vi "driveForwardFast Command.vi"(10 "Data":string[](array[string]), 11 "Robot dev revs":T1={"Drive"={"Drive Actuaters"={"Motor devRevs"={"Left Side Motors"={"Motor 1 devRev"={"DeviceStatus"={"status"=FALSE, "code"=0, "source"=""}, "Type"=enum."PWM", "PWM"={"Digital Module"=enum."Digital Module 1", "PWM Channel"=enum."PWM 1", "DeadBand"={"Name"="", "maxPositivePwm"=0, "minPositivePwm"=0, "centerPwm"=0, "maxNegativePwm"=0, "minNegativePwm"=0, "angularRange"=0}}, "CAN"={"Device Number"=0, "Control Mode"=enum."Percent VBus", "Semaphore"=refnum, "Max Vout"=0.0}, "Invert"=FALSE, "TransformRef"=refnum, "InvTransformRef"=refnum}, "Motor 2 devRev"={"DeviceStatus"={"status"=FALSE, "code"=0, "source"=""}, "Type"=enum."PWM", "PWM"={"Digital Module"=enum."Digital Module 1", "PWM Channel"=enum."PWM 1", "DeadBand"={"Name"="", "maxPositivePwm"=0, "minPositivePwm"=0, "centerPwm"=0, "maxNegativePwm"=0, "minNegativePwm"=0, "angularRange"=0}}, "CAN"={"Device Number"=0, "Control Mode"=enum."Percent VBus", "Semaphore"=refnum, "Max Vout"=0.0}, "Invert"=FALSE, "TransformRef"=refnum, "InvTransformRef"=refnum}, "Motor 3 devRev"={"DeviceStatus"={"status"=FALSE, "code"=0, "source"=""}, "Type"=enum."PWM", "PWM"={"Digital Module"=enum."Digital Module 1", "PWM Channel"=enum."PWM 1", "DeadBand"={"Name"="", "maxPositivePwm"=0, "minPositivePwm"=0, "centerPwm"=0, "maxNegativePwm"=0, "minNegativePwm"=0, "angularRange"=0}}, "CAN"={"Device Number"=0, "Control Mode"=enum."Percent VBus", "Semaphore"=refnum, "Max Vout"=0.0}, "Invert"=FALSE, "TransformRef"=refnum, "InvTransformRef"=refnum}}, "Right Side Motors"={"Motor 1 devRev"={"DeviceStatus"={"status"=FALSE, "code"=0, "source"=""}, "Type"=enum."PWM", "PWM"={"Digital Module"=enum."Digital Module 1", "PWM Channel"=enum."PWM 1", "DeadBand"={"Name"="", "maxPositivePwm"=0, "minPositivePwm"=0, "centerPwm"=0, "maxNegativePwm"=0, "minNegativePwm"=0, "angularRange"=0}}, "CAN"={"Device Number"=0, "Control Mode"=enum."Percent VBus", "Semaphore"=refnum, "Max Vout"=0.0}, "Invert"=FALSE, "TransformRef"=refnum, "InvTransformRef"=refnum}, "Motor 2 devRev"={"DeviceStatus"={"status"=FALSE, "code"=0, "source"=""}, "Type"=enum."PWM", "PWM"={"Digital Module"=enum."Digital Module 1", "PWM Channel"=enum."PWM 1", "DeadBand"={"Name"="", "maxPositivePwm"=0, "minPositivePwm"=0, "centerPwm"=0, "maxNegativePwm"=0, "minNegativePwm"=0, "angularRange"=0}}, "CAN"={"Device Number"=0, "Control Mode"=enum."Percent VBus", "Semaphore"=refnum, "Max Vout"=0.0}, "Invert"=FALSE, "TransformRef"=refnum, "InvTransformRef"=refnum}, "Motor 3 devRev"={"DeviceStatus"={"status"=FALSE, "code"=0, "source"=""}, "Type"=enum."PWM", "PWM"={"Digital Module"=enum."Digital Module 1", "PWM Channel"=enum."PWM 1", "DeadBand"={"Name"="", "maxPositivePwm"=0, "minPositivePwm"=0, "centerPwm"=0, "maxNegativePwm"=0, "minNegativePwm"=0, "angularRange"=0}}, "CAN"={"Device Number"=0, "Control Mode"=enum."Percent VBus", "Semaphore"=refnum, "Max Vout"=0.0}, "Invert"=FALSE, "TransformRef"=refnum, "InvTransformRef"=refnum}}, "dev Status"={"status"=FALSE, "code"=0, "source"=""}}, "SolenoidDevRef"={"DevStatus"={"status"=FALSE, "code"=0, "source"=""}, "Solenoid Module"=enum."Solenoid Module 1", "Forward Solenoid Channel"=enum."Solenoid 1", "Reverse Solenoid Channel"=enum."Solenoid 1"}}, "Drive Sensor data"={"Encoders"={"Right Encoder"={"DevStatus"={"status"=FALSE, "code"=0, "source"=""}, "EncoderIndex"=enum."Enc 0", "CounterIndex"=enum."Ctr 0", "DistancePerCount"=0.0, "Decoding Type"=enum."1x"}}, "GyroDevRef"={"DevStatus"={"status"=FALSE, "code"=0, "source"=""}, "Analog Module"=enum."Analog Module 1", "Analog Channel"=enum."AI 1", "Offset"=0.0, "Gain (VoltsPerDegree/Second)"=0.0}, "Last commanded Angle"=0.0}}, "Catapult devrevs"={"MotorControlDeviceRef"={"DeviceStatus"={"status"=FALSE, "code"=0, "source"=""}, "Type"=enum."PWM", "PWM"={"Digital Module"=enum."Digital Module 1", "PWM Channel"=enum."PWM 1", "DeadBand"={"Name"="", "maxPositivePwm"=0, "minPositivePwm"=0, "centerPwm"=0, "maxNegativePwm"=0, "minNegativePwm"=0, "angularRange"=0}}, "CAN"={"Device Number"=0, "Control Mode"=enum."Percent VBus", "Semaphore"=refnum, "Max Vout"=0.0}, "Invert"=FALSE, "TransformRef"=refnum, "InvTransformRef"=refnum}, "SolenoidDevRef"={"DevStatus"={"status"=FALSE, "code"=0, "source"=""}, "Solenoid Module"=enum."Solenoid Module 1", "Forward Solenoid Channel"=enum."Solenoid 1", "Reverse Solenoid Channel"=enum."Solenoid 1"}, "first limit switch"={"DevStatus"={"status"=FALSE, "code"=0, "source"=""}, "DIO Channel"=enum."DIO 1", "Digital Module"=enum."Digital Module 1"}, "second limit switch"={"DevStatus"={"status"=FALSE, "code"=0, "source"=""}, "DIO Channel"=enum."DIO 1", "Digital Module"=enum."Digital Module 1"}}, "Drive Joystick"={"Device"=enum."USB 1"}, "Operator Joystick"={"Device"=enum."USB 1"}, "roller devrevs"={"SolenoidDevRef"={"DevStatus"={"status"=FALSE, "code"=0, "source"=""}, "Solenoid Module"=enum."Solenoid Module 1", "Forward Solenoid Channel"=enum."Solenoid 1", "Reverse Solenoid Channel"=enum."Solenoid 1"}, "MotorControlDeviceRef"={"DeviceStatus"={"status"=FALSE, "code"=0, "source"=""}, "Type"=enum."PWM", "PWM"={"Digital Module"=enum."Digital Module 1", "PWM Channel"=enum."PWM 1", "DeadBand"={"Name"="", "maxPositivePwm"=0, "minPositivePwm"=0, "centerPwm"=0, "maxNegativePwm"=0, "minNegativePwm"=0, "angularRange"=0}}, "CAN"={"Device Number"=0, "Control Mode"=enum."Percent VBus", "Semaphore"=refnum, "Max Vout"=0.0}, "Invert"=FALSE, "TransformRef"=refnum, "InvTransformRef"=refnum}, "DigitalInputDevRef"={"DevStatus"={"status"=FALSE, "code"=0, "source"=""}, "DIO Channel"=enum."Invalid", "Digital Module"=enum."Digital Module 1"}}, "Puncher devrevs"={"SolenoidDevRef"={"DevStatus"={"status"=FALSE, "code"=0, "source"=""}, "Solenoid Module"=enum."Solenoid Module 1", "Forward Solenoid Channel"=enum."Solenoid 1", "Reverse Solenoid Channel"=enum."Solenoid 1"}, "DigitalInputDevRef"={"DevStatus"={"status"=FALSE, "code"=0, "source"=""}, "DIO Channel"=enum."DIO 1", "Digital Module"=enum."Digital Module 1"}}}) -> (3 "Robot dev revs out":T1={"Drive"={"Drive Actuaters"={"Motor devRevs"={"Left Side Motors"={"Motor 1 devRev"={"DeviceStatus"={"status"=FALSE, "code"=0, "source"=""}, "Type"=enum."PWM", "PWM"={"Digital Module"=enum."Digital Module 1", "PWM Channel"=enum."PWM 1", "DeadBand"={"Name"="", "maxPositivePwm"=0, "minPositivePwm"=0, "centerPwm"=0, "maxNegativePwm"=0, "minNegativePwm"=0, "angularRange"=0}}, "CAN"={"Device Number"=0, "Control Mode"=enum."Percent VBus", "Semaphore"=refnum, "Max Vout"=0.0}, "Invert"=FALSE, "TransformRef"=refnum, "InvTransformRef"=refnum}, "Motor 2 devRev"={"DeviceStatus"={"status"=FALSE, "code"=0, "source"=""}, "Type"=enum."PWM", "PWM"={"Digital Module"=enum."Digital Module 1", "PWM Channel"=enum."PWM 1", "DeadBand"={"Name"="", "maxPositivePwm"=0, "minPositivePwm"=0, "centerPwm"=0, "maxNegativePwm"=0, "minNegativePwm"=0, "angularRange"=0}}, "CAN"={"Device Number"=0, "Control Mode"=enum."Percent VBus", "Semaphore"=refnum, "Max Vout"=0.0}, "Invert"=FALSE, "TransformRef"=refnum, "InvTransformRef"=refnum}, "Motor 3 devRev"={"DeviceStatus"={"status"=FALSE, "code"=0, "source"=""}, "Type"=enum."PWM", "PWM"={"Digital Module"=enum."Digital Module 1", "PWM Channel"=enum."PWM 1", "DeadBand"={"Name"="", "maxPositivePwm"=0, "minPositivePwm"=0, "centerPwm"=0, "maxNegativePwm"=0, "minNegativePwm"=0, "angularRange"=0}}, "CAN"={"Device Number"=0, "Control Mode"=enum."Percent VBus", "Semaphore"=refnum, "Max Vout"=0.0}, "Invert"=FALSE, "TransformRef"=refnum, "InvTransformRef"=refnum}}, "Right Side Motors"={"Motor 1 devRev"={"DeviceStatus"={"status"=FALSE, "code"=0, "source"=""}, "Type"=enum."PWM", "PWM"={"Digital Module"=enum."Digital Module 1", "PWM Channel"=enum."PWM 1", "DeadBand"={"Name"="", "maxPositivePwm"=0, "minPositivePwm"=0, "centerPwm"=0, "maxNegativePwm"=0, "minNegativePwm"=0, "angularRange"=0}}, "CAN"={"Device Number"=0, "Control Mode"=enum."Percent VBus", "Semaphore"=refnum, "Max Vout"=0.0}, "Invert"=FALSE, "TransformRef"=refnum, "InvTransformRef"=refnum}, "Motor 2 devRev"={"DeviceStatus"={"status"=FALSE, "code"=0, "source"=""}, "Type"=enum."PWM", "PWM"={"Digital Module"=enum."Digital Module 1", "PWM Channel"=enum."PWM 1", "DeadBand"={"Name"="", "maxPositivePwm"=0, "minPositivePwm"=0, "centerPwm"=0, "maxNegativePwm"=0, "minNegativePwm"=0, "angularRange"=0}}, "CAN"={"Device Number"=0, "Control Mode"=enum."Percent VBus", "Semaphore"=refnum, "Max Vout"=0.0}, "Invert"=FALSE, "TransformRef"=refnum, "InvTransformRef"=refnum}, "Motor 3 devRev"={"DeviceStatus"={"status"=FALSE, "code"=0, "source"=""}, "Type"=enum."PWM", "PWM"={"Digital Module"=enum."Digital Module 1", "PWM Channel"=enum."PWM 1", "DeadBand"={"Name"="", "maxPositivePwm"=0, "minPositivePwm"=0, "centerPwm"=0, "maxNegativePwm"=0, "minNegativePwm"=0, "angularRange"=0}}, "CAN"={"Device Number"=0, "Control Mode"=enum."Percent VBus", "Semaphore"=refnum, "Max Vout"=0.0}, "Invert"=FALSE, "TransformRef"=refnum, "InvTransformRef"=refnum}}, "dev Status"={"status"=FALSE, "code"=0, "source"=""}}, "SolenoidDevRef"={"DevStatus"={"status"=FALSE, "code"=0, "source"=""}, "Solenoid Module"=enum."Solenoid Module 1", "Forward Solenoid Channel"=enum."Solenoid 1", "Reverse Solenoid Channel"=enum."Solenoid 1"}}, "Drive Sensor data"={"Encoders"={"Right Encoder"={"DevStatus"={"status"=FALSE, "code"=0, "source"=""}, "EncoderIndex"=enum."Enc 0", "CounterIndex"=enum."Ctr 0", "DistancePerCount"=0.0, "Decoding Type"=enum."1x"}}, "GyroDevRef"={"DevStatus"={"status"=FALSE, "code"=0, "source"=""}, "Analog Module"=enum."Analog Module 1", "Analog Channel"=enum."AI 1", "Offset"=0.0, "Gain (VoltsPerDegree/Second)"=0.0}, "Last commanded Angle"=0.0}}, "Catapult devrevs"={"MotorControlDeviceRef"={"DeviceStatus"={"status"=FALSE, "code"=0, "source"=""}, "Type"=enum."PWM", "PWM"={"Digital Module"=enum."Digital Module 1", "PWM Channel"=enum."PWM 1", "DeadBand"={"Name"="", "maxPositivePwm"=0, "minPositivePwm"=0, "centerPwm"=0, "maxNegativePwm"=0, "minNegativePwm"=0, "angularRange"=0}}, "CAN"={"Device Number"=0, "Control Mode"=enum."Percent VBus", "Semaphore"=refnum, "Max Vout"=0.0}, "Invert"=FALSE, "TransformRef"=refnum, "InvTransformRef"=refnum}, "SolenoidDevRef"={"DevStatus"={"status"=FALSE, "code"=0, "source"=""}, "Solenoid Module"=enum."Solenoid Module 1", "Forward Solenoid Channel"=enum."Solenoid 1", "Reverse Solenoid Channel"=enum."Solenoid 1"}, "first limit switch"={"DevStatus"={"status"=FALSE, "code"=0, "source"=""}, "DIO Channel"=enum."DIO 1", "Digital Module"=enum."Digital Module 1"}, "second limit switch"={"DevStatus"={"status"=FALSE, "code"=0, "source"=""}, "DIO Channel"=enum."DIO 1", "Digital Module"=enum."Digital Module 1"}}, "Drive Joystick"={"Device"=enum."USB 1"}, "Operator Joystick"={"Device"=enum."USB 1"}, "roller devrevs"={"SolenoidDevRef"={"DevStatus"={"status"=FALSE, "code"=0, "source"=""}, "Solenoid Module"=enum."Solenoid Module 1", "Forward Solenoid Channel"=enum."Solenoid 1", "Reverse Solenoid Channel"=enum."Solenoid 1"}, "MotorControlDeviceRef"={"DeviceStatus"={"status"=FALSE, "code"=0, "source"=""}, "Type"=enum."PWM", "PWM"={"Digital Module"=enum."Digital Module 1", "PWM Channel"=enum."PWM 1", "DeadBand"={"Name"="", "maxPositivePwm"=0, "minPositivePwm"=0, "centerPwm"=0, "maxNegativePwm"=0, "minNegativePwm"=0, "angularRange"=0}}, "CAN"={"Device Number"=0, "Control Mode"=enum."Percent VBus", "Semaphore"=refnum, "Max Vout"=0.0}, "Invert"=FALSE, "TransformRef"=refnum, "InvTransformRef"=refnum}, "DigitalInputDevRef"={"DevStatus"={"status"=FALSE, "code"=0, "source"=""}, "DIO Channel"=enum."Invalid", "Digital Module"=enum."Digital Module 1"}}, "Puncher devrevs"={"SolenoidDevRef"={"DevStatus"={"status"=FALSE, "code"=0, "source"=""}, "Solenoid Module"=enum."Solenoid Module 1", "Forward Solenoid Channel"=enum."Solenoid 1", "Reverse Solenoid Channel"=enum."Solenoid 1"}, "DigitalInputDevRef"={"DevStatus"={"status"=FALSE, "code"=0, "source"=""}, "DIO Channel"=enum."DIO 1", "Digital Module"=enum."Digital Module 1"}}})   [LabVIEW 2013]
uses:
  Robot dev revs.ctl
  Drive Code/Drive typedef.ctl
  Drive Code/Drive Motors Typedef.ctl
  Drive Code/GearBox Typedef.ctl
  <vilib>/Rock Robotics/WPI/MotorControl/WPI_MotorControlDeviceRef.ctl
  <vilib>/Rock Robotics/SystemInterfaces/Typedef/FPGA_TypedefDigitalModule.ctl
  <vilib>/Rock Robotics/SystemInterfaces/DIO/FPGA_DIOPWMChannel.ctl
  <vilib>/Rock Robotics/WPI/PWM/WPI_PWMDeadband.ctl
  <vilib>/Rock Robotics/WPI/CAN/Jaguar/SubVIs/WPI_CANJaguar_ControlMode.ctl
  <vilib>/Rock Robotics/WPI/PWM/WPI_PWMTransform_ConPane.ctl
  <vilib>/Rock Robotics/WPI/Solenoid/WPI_SolenoidDevRef.ctl
  <vilib>/Rock Robotics/SystemInterfaces/Typedef/FPGA_TypedefSolenoidModule.ctl
  <vilib>/Rock Robotics/WPI/Solenoid/WPI_SolenoidChannel.ctl
  Drive Code/Drive Sensor Typedef.ctl
  <vilib>/Rock Robotics/WPI/Encoder/WPI_EncoderDevRef.ctl
  <vilib>/Rock Robotics/SystemInterfaces/Encoder/FPGA_EncoderIdx.ctl
  <vilib>/Rock Robotics/SystemInterfaces/Counter/FPGA_CounterCtrSystemIndex.ctl
  <vilib>/Rock Robotics/WPI/Encoder/WPI_EncoderType.ctl
  <vilib>/Rock Robotics/WPI/Gyro/WPI_GyroDevRef.ctl
  <vilib>/Rock Robotics/SystemInterfaces/Typedef/FPGA_TypedefAnalogModule.ctl
  <vilib>/Rock Robotics/SystemInterfaces/AI/FPGA_AIChannel.ctl
  catapult code/catapult type def.ctl
  <vilib>/Rock Robotics/WPI/DigitalInput/WPI_DigitalInputDevRef.ctl
  <vilib>/Rock Robotics/SystemInterfaces/DIO/FPGA_DIOChannel.ctl
  <vilib>/Rock Robotics/WPI/Joystick/WPI_JoystickDevRef.ctl
  <vilib>/Rock Robotics/WPI/Joystick/WPI_JoystickDeviceEnum.ctl
  Roller V2/roller typedef.ctl
  Puncher/Puncher type.ctl
  Drive Auto/All Auto Drive constants.ctl
  Drive Auto/Drive auto constants.ctl
  Drive Code/Auto Transmission Code/All Shifter Constants.ctl
  Drive Code/Auto Transmission Code/Shift Constants.ctl
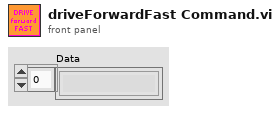
[diagram p1: front panel]
types:
  T1 = typedef "Robot dev revs.ctl" = cluster{"Drive":T2, "Catapult devrevs":T23, "Drive Joystick":T26, "Operator Joystick":T26, "roller devrevs":T28, "Puncher devrevs":T29}
  T2 = typedef "Drive typedef.ctl" = cluster{"Drive Actuaters":cluster{"Motor devRevs":T3, "SolenoidDevRef":T12}, "Drive Sensor data":T15}
  T3 = typedef "Drive Motors Typedef.ctl" = cluster{"Left Side Motors":T4, "Right Side Motors":T4, "dev Status":errorcluster}
  T4 = typedef "GearBox Typedef.ctl" = cluster{"Motor 1 devRev":T5, "Motor 2 devRev":T5, "Motor 3 devRev":T5}
  T5 = typedef "WPI_MotorControlDeviceRef.ctl" = cluster{"DeviceStatus":errorcluster, "Type":enum16{"PWM", "CAN"}, "PWM":cluster{"Digital Module":T6, "PWM Channel":T7, "DeadBand":T8}, "CAN":cluster{"Device Number":u8, "Control Mode":T9, "Semaphore":T10, "Max Vout":dbl}, "Invert":bool, "TransformRef":T11, "InvTransformRef":T11}
  T6 = typedef "FPGA_TypedefDigitalModule.ctl" = enum16{"Digital Module 1", "Digital Module 2"}
  T7 = typedef "FPGA_DIOPWMChannel.ctl" = enum8{"PWM 1", "PWM 2", "PWM 3", "PWM 4", "PWM 5", "PWM 6", "PWM 7", "PWM 8", "PWM 9", "PWM 10", "Invalid"}
  T8 = typedef "WPI_PWMDeadband.ctl" = cluster{"Name":string, "maxPositivePwm":i32, "minPositivePwm":i32, "centerPwm":i32, "maxNegativePwm":i32, "minNegativePwm":i32, "angularRange":u16}
  T9 = typedef "WPI_CANJaguar_ControlMode.ctl" = enum8{"Percent VBus", "Current", "Speed", "Position", "Voltage"}
  T10 = typedef "Semaphore RefNum" = refnum<k1>
  T11 = typedef "WPI_PWMTransform_ConPane.ctl" = refnum<vi>
  T12 = typedef "WPI_SolenoidDevRef.ctl" = cluster{"DevStatus":errorcluster, "Solenoid Module":T13, "Forward Solenoid Channel":T14, "Reverse Solenoid Channel":T14}
  T13 = typedef "FPGA_TypedefSolenoidModule.ctl" = enum16{"Solenoid Module 1", "Solenoid Module 2"}
  T14 = typedef "WPI_SolenoidChannel.ctl" = enum8{"Solenoid 1", "Solenoid 2", "Solenoid 3", "Solenoid 4", "Solenoid 5", "Solenoid 6", "Solenoid 7", "Solenoid 8", "Invalid"}
  T15 = typedef "Drive Sensor Typedef.ctl" = cluster{"Encoders":cluster{"Right Encoder":T16}, "GyroDevRef":T20, "Last commanded Angle":dbl}
  T16 = typedef "WPI_EncoderDevRef.ctl" = cluster{"DevStatus":errorcluster, "EncoderIndex":T17, "CounterIndex":T18, "DistancePerCount":dbl, "Decoding Type":T19}
  T17 = typedef "FPGA_EncoderIdx.ctl" = enum8{"Enc 0", "Enc 1", "Enc 2", "Enc 3", "Invalid"}
  T18 = typedef "FPGA_CounterCtrSystemIndex.ctl" = enum8{"Ctr 0", "Ctr 1", "Ctr 2", "Ctr 3", "Ctr 4", "Ctr 5", "Ctr 6", "Ctr 7", "Invalid"}
  T19 = typedef "WPI_EncoderType.ctl" = enum16{"1x", "2x", "4x"}
  T20 = typedef "WPI_GyroDevRef.ctl" = cluster{"DevStatus":errorcluster, "Analog Module":T21, "Analog Channel":T22, "Offset":dbl, "Gain (VoltsPerDegree/Second)":dbl}
  T21 = typedef "FPGA_TypedefAnalogModule.ctl" = enum16{"Analog Module 1", "Analog Module 2"}
  T22 = typedef "FPGA_AIChannel.ctl" = enum8{"AI 1", "AI 2", "AI 3", "AI 4", "AI 5", "AI 6", "AI 7", "AI 8", "Invalid"}
  T23 = typedef "catapult type def.ctl" = cluster{"MotorControlDeviceRef":T5, "SolenoidDevRef":T12, "first limit switch":T24, "second limit switch":T24}
  T24 = typedef "WPI_DigitalInputDevRef.ctl" = cluster{"DevStatus":errorcluster, "DIO Channel":T25, "Digital Module":T6}
  T25 = typedef "FPGA_DIOChannel.ctl" = enum8{"DIO 1", "DIO 2", "DIO 3", "DIO 4", "DIO 5", "DIO 6", "DIO 7", "DIO 8", "DIO 9", "DIO 10", "DIO 11", "DIO 12", "DIO 13", "DIO 14", "Invalid"}
  T26 = typedef "WPI_JoystickDevRef.ctl" = cluster{"Device":T27}
  T27 = typedef "WPI_JoystickDeviceEnum.ctl" = enum16{"USB 1", "USB 2", "USB 3", "USB 4", "Kinect 1", "Kinect 2"}
  T28 = typedef "roller typedef.ctl" = cluster{"SolenoidDevRef":T12, "MotorControlDeviceRef":T5, "DigitalInputDevRef":T24}
  T29 = typedef "Puncher type.ctl" = cluster{"SolenoidDevRef":T12, "DigitalInputDevRef":T24}
  T30 = typedef "All Auto Drive constants.ctl" = cluster{"Drive auto Constants":T31, "All Shifter Constants":T32}
  T31 = typedef "Drive auto constants.ctl" = cluster{"PID Gains":cluster{"High Gear Gains":cluster{"PID Turn Gains":cluster{"proportional gain (Kc)":dbl, "integral time (Ti, min)":dbl, "derivative time (Td, min)":dbl}, "PID Straight Gains":cluster{"proportional gain (Kc)":dbl, "integral time (Ti, min)":dbl, "derivative time (Td, min)":dbl}}, "Low Gains":cluster{"PID Turn Gains":cluster{"proportional gain (Kc)":dbl, "integral time (Ti, min)":dbl, "derivative time (Td, min)":dbl}, "PID Straight Gains":cluster{"proportional gain (Kc)":dbl, "integral time (Ti, min)":dbl, "derivative time (Td, min)":dbl}}}, "Deadbands":cluster{"Turn Deadband":dbl, "Straight Deadband":dbl, "Mili seconds to wait to in deadband":u32}}
  T32 = typedef "All Shifter Constants.ctl" = cluster{"Drive info constants":cluster{"Enocder Pulses per foot":dbl, "Amount of turn before drive is turning":dbl}, "Shift control Constants":T33}
  T33 = typedef "Shift Constants.ctl" = cluster{"Global shift constants":cluster{"Mili seconds before it can shift again":u32, "Max fps":dbl}, "Upshift constants":cluster{"Upshift point in fps":dbl, "Upshift Accel constant":dbl, "Commanded Throttle  shiftpoint gain":dbl}, "Downshift Constants":cluster{"Kickdown shift point":dbl, "Kickdown at -acceleration":dbl, "Slowest Throttle for kickdown":dbl, "Coastdown shift speed":dbl}}
  T34 = cluster{"Forced high gear?":bool, "Force which gear it is in":bool}
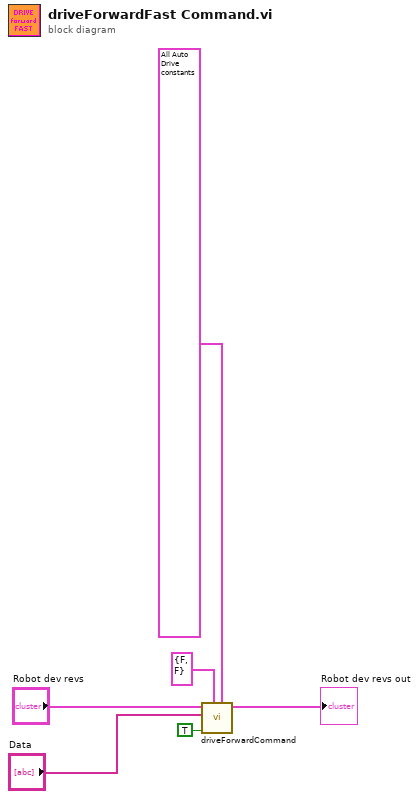
[diagram p0: block diagram]
diagram:
  n1 = call "driveForwardCommand.vi"("All Auto Drive constants"=T30 {"Drive auto Constants"={"PID Gains"={"High Gear Gains"={"PID Turn Gains"={"proportional gain (Kc)"=0.0, "integral time (Ti, min)"=0.0, "derivative time (Td, min)"=0.0}, "PID Straight Gains"={"proportional gain (Kc)"=0.0, "integral time (Ti, min)"=0.0, "derivative time (Td, min)"=0.0}}, "Low Gains"={"PID Turn Gains"={"proportional gain (Kc)"=0.0, "integral time (Ti, min)"=0.0, "derivative time (Td, min)"=0.0}, "PID Straight Gains"={"proportional gain (Kc)"=0.0, "integral time (Ti, min)"=0.0, "derivative time (Td, min)"=0.0}}}, "Deadbands"={"Turn Deadband"=0.0, "Straight Deadband"=0.0, "Mili seconds to wait to in deadband"=0}}, "All Shifter Constants"={"Drive info constants"={"Enocder Pulses per foot"=0.0, "Amount of turn before drive is turning"=0.0}, "Shift control Constants"={"Global shift constants"={"Mili seconds before it can shift again"=0, "Max fps"=0.0}, "Upshift constants"={"Upshift point in fps"=0.0, "Upshift Accel constant"=0.0, "Commanded Throttle  shiftpoint gain"=0.0}, "Downshift Constants"={"Kickdown shift point"=0.0, "Kickdown at -acceleration"=0.0, "Slowest Throttle for kickdown"=0.0, "Coastdown shift speed"=0.0}}}}, "Shifting controls"=T34 {"Forced high gear?"=FALSE, "Force which gear it is in"=FALSE}, "Quick stop"=TRUE, "Data"="Data", "Robot dev revs"="Robot dev revs") -> ("Robot dev revs"=→"Robot dev revs out":T1)  [unwired: 6 in]
